vi "SUMMER SUNDAY BYTE[1].vi"() -> ()   [LabVIEW 2009]
uses:
  <vilib>/ULx/Create Channel.llb/ULx Create Channel (AI-Voltage-Basic).vi
  <vilib>/ULx/Read.llb/ULx Read (Analog DBL 1Chan 1Samp).vi
panel:
  out "POWER":bool
  out "data":dbl format="%_6g"
  out "xray":bool caption="BitValue"
  out "ENERGY LEVEL":dbl(knob) scale=0.0..15.0
  out "x*y":dbl
  out "Beam Pot":dbl format="%_6g"
  out "READY 2":bool
  out "DUMP":bool
  out "POWER":bool
  out "?":bool
  out "?":bool
  out "?":bool
  out "?":bool
  out "?":bool
  out "?":bool
  out "?":bool
  out "?":bool
  out "?":bool
  out "?":bool
  out "OPEN":bool
  out "CLOSED":bool
  out "READY":bool
  out "FAULT":bool
  out "MAGNET FORCE":dbl(slide) scale=0.0..10.0
  out "READY":bool
  out "TEMPERATURE":dbl(slide) scale=0.0..10.0
  in  "stop":bool
  out "?":bool
  out "?":bool
  out "?":bool
  out "?":bool
  in  "FAULT":bool
  out "POWER":bool
  out "FLOW IN GPM":dbl(knob) scale=0.0..15.0
  # "USERS LAB AREA"
  # "BEAM STATUS"
  # "ROOM"
  # "XRAY"
  # "PUMP STATION"
  # "MAGNET STATUS"
  # "ORBIT"
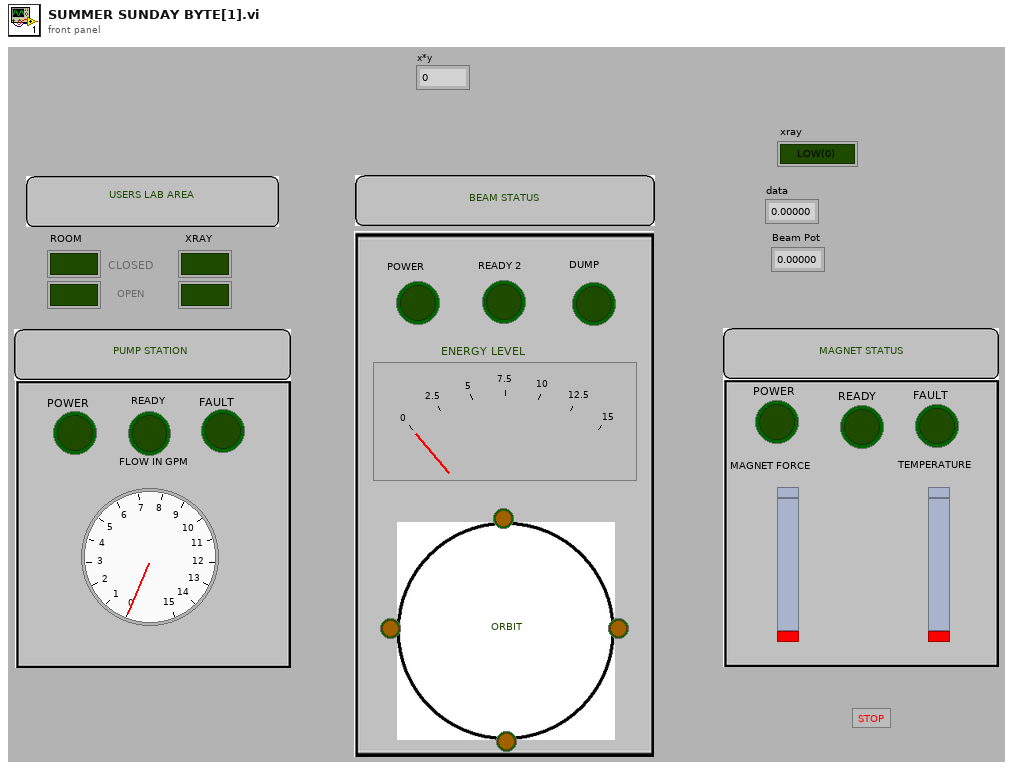
[diagram p1: front panel]
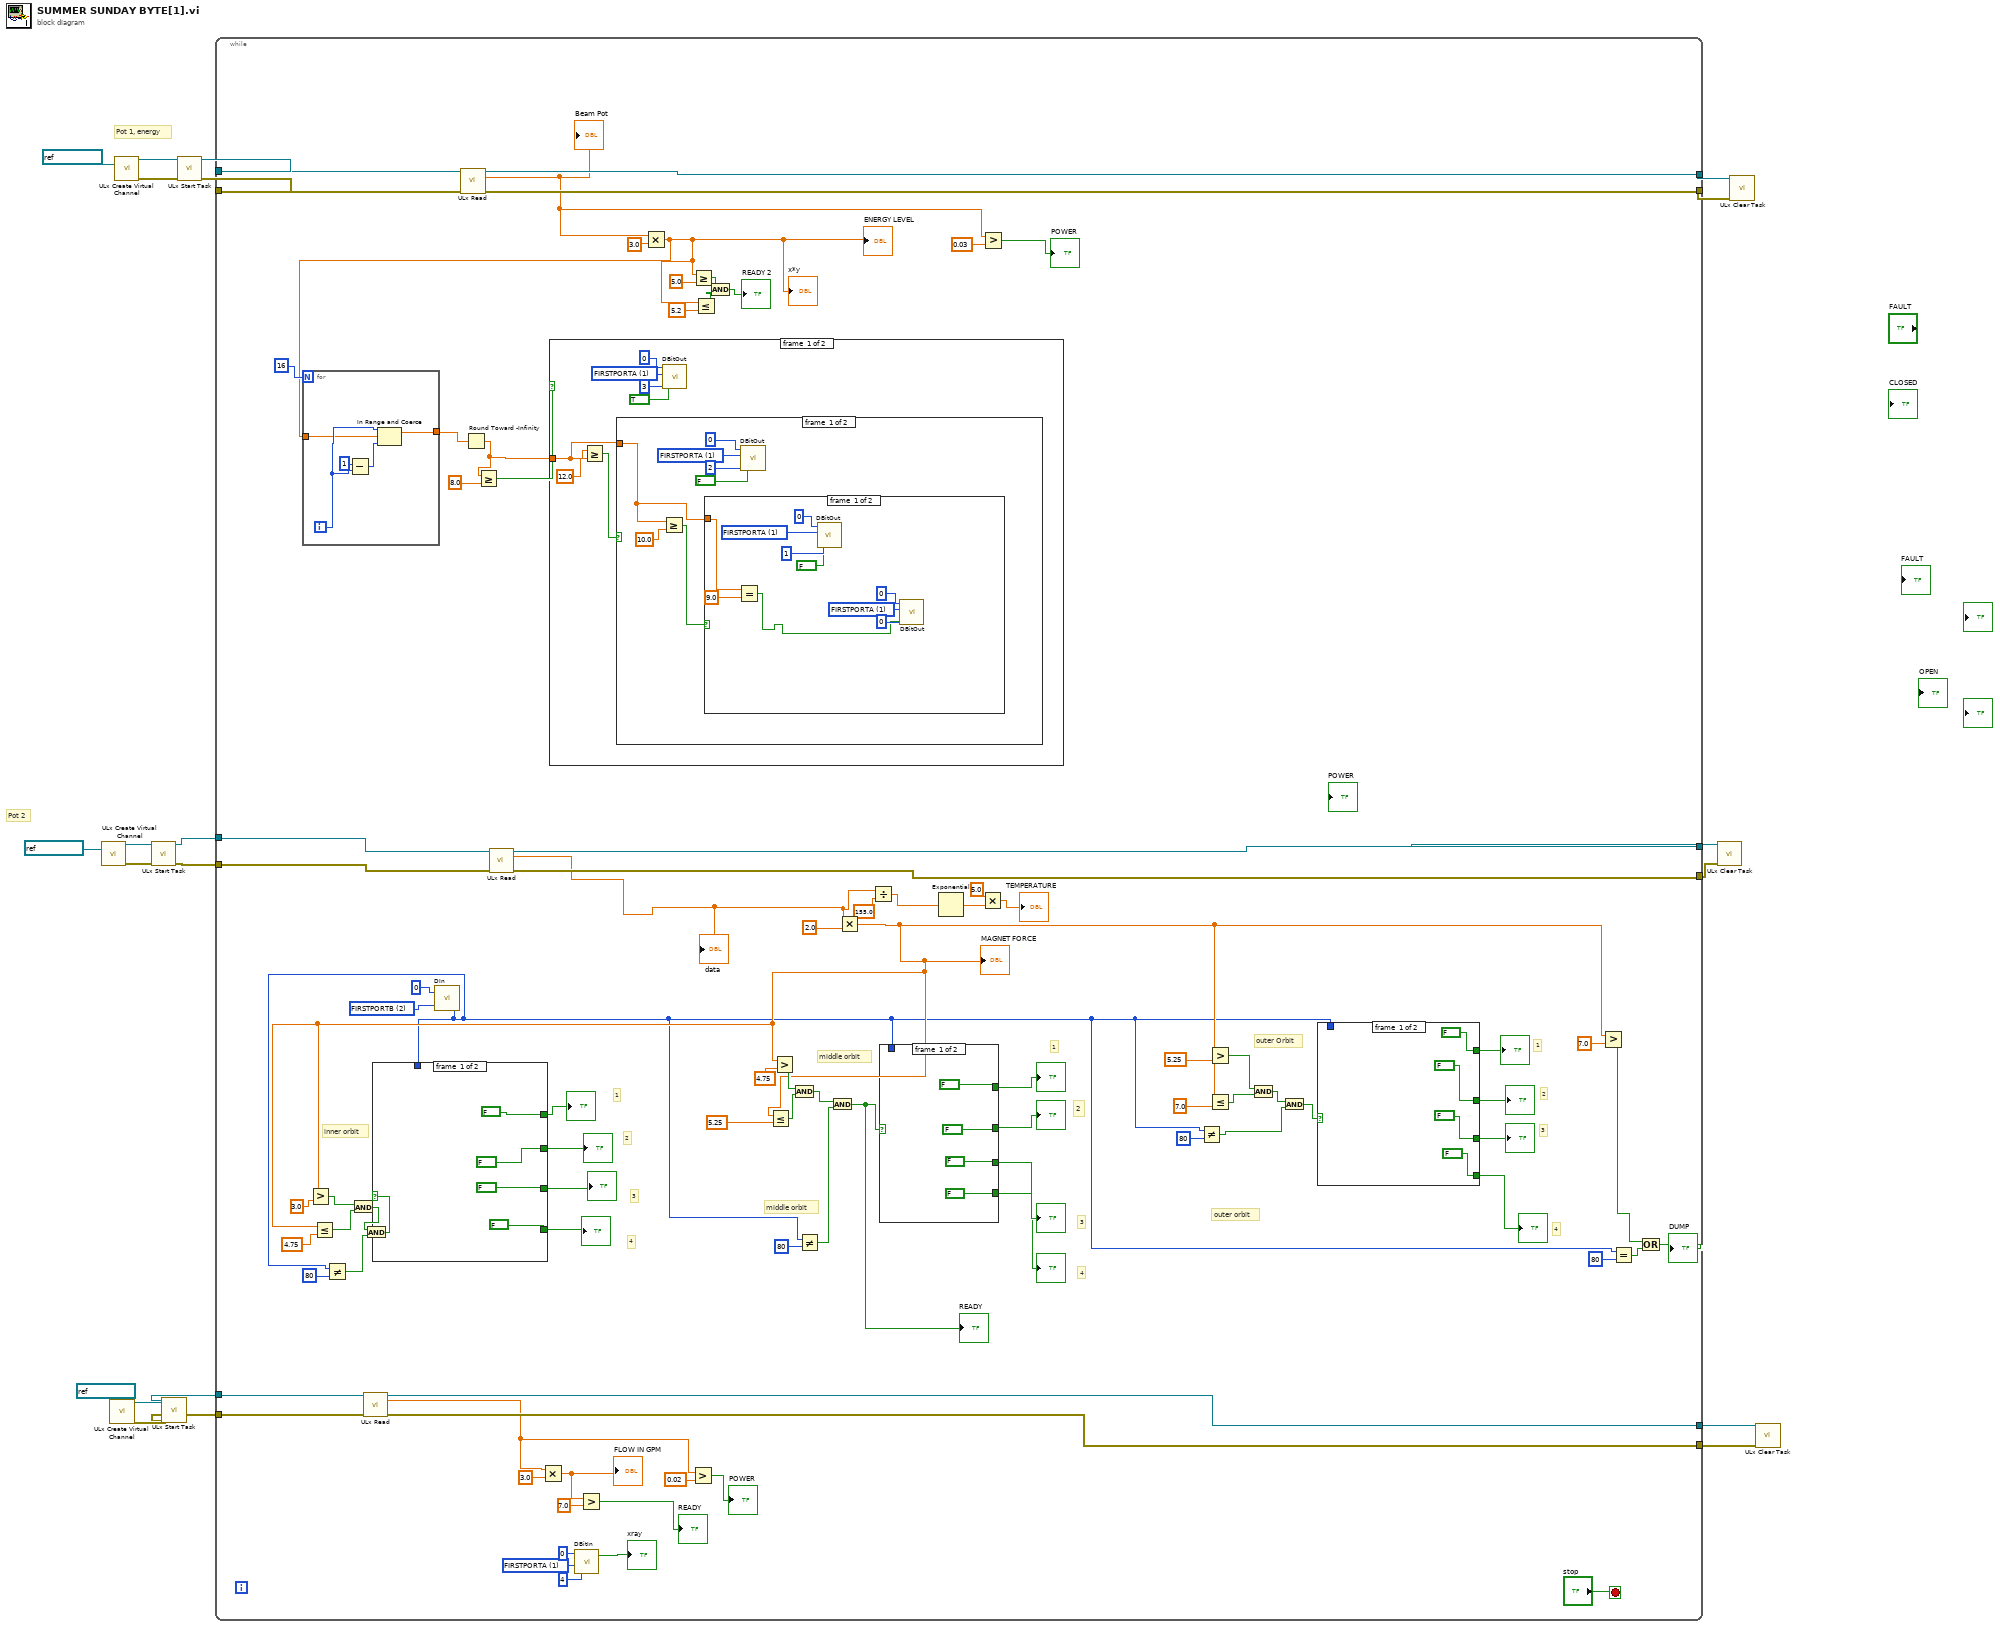
[diagram p0: block diagram]
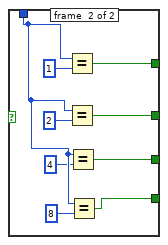
[diagram p2: hidden frame]
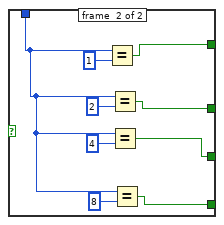
[diagram p3: hidden frame]
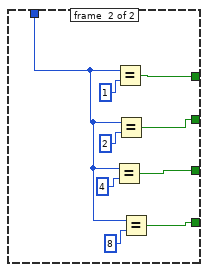
[diagram p4: hidden frame]
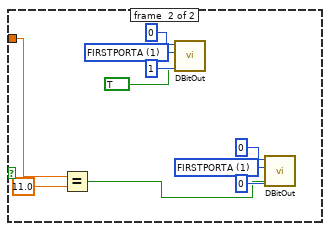
[diagram p5: hidden frame]
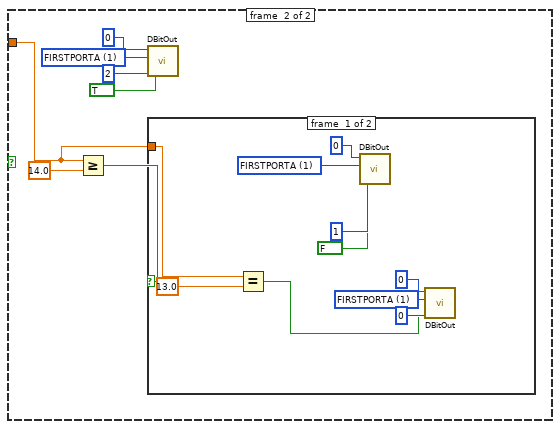
[diagram p6: hidden frame]
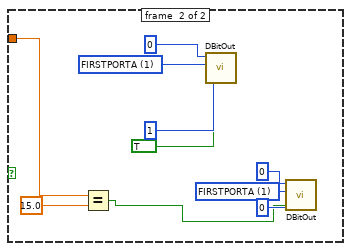
[diagram p7: hidden frame]
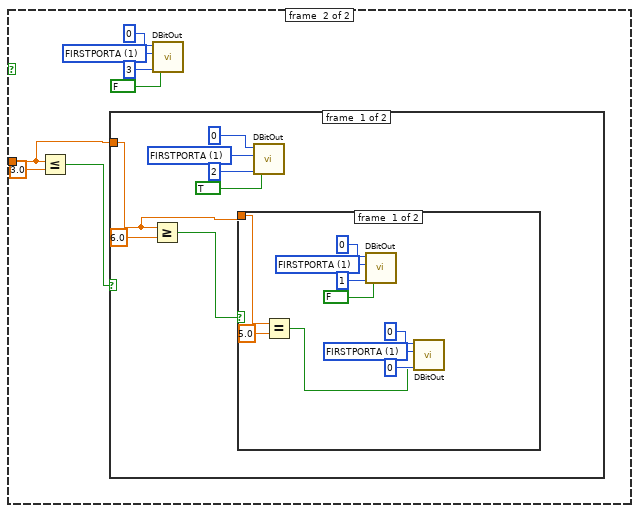
[diagram p8: hidden frame]
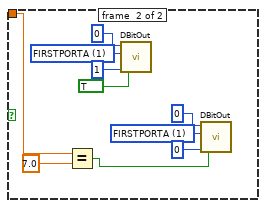
[diagram p9: hidden frame]
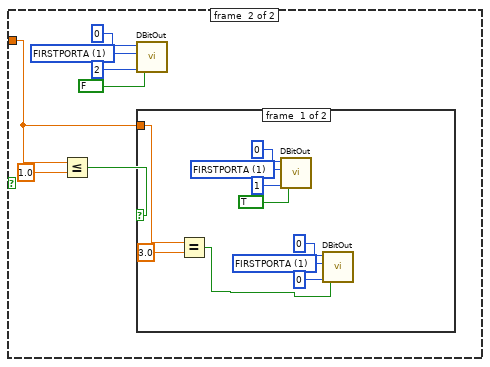
[diagram p10: hidden frame]
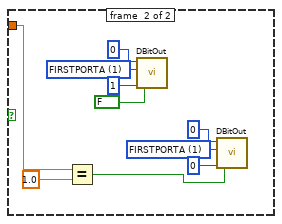
[diagram p11: hidden frame]
diagram:
  # "Pot 2"
  # "Pot 1, energy"
  n1 = call-poly <vilib>:"ULx Create Virtual Channel.vi"("physical channels"=refnum<k21> "Dev0/Ai1") -> ("task out"=w15:refnum<k24>, "error out"=w14:errorcluster)  [unwired: 13 in]
  n2 = call-poly <vilib>:"ULx Create Virtual Channel.vi"("physical channels"=refnum<k21> "Dev0/Ai2") -> ("task out"=w7:refnum<k24>, "error out"=w6:errorcluster)  [unwired: 13 in]
  n3 = call-poly <vilib>:"ULx Create Virtual Channel.vi"("physical channels"=refnum<k21> "Dev0/Ai0") -> ("task out"=w21:refnum<k24>, "error out"=w20:errorcluster)  [unwired: 13 in]
  n4 = call <vilib>:"ULx Start Task.vi"("task in"=w15, "error in"=w14) -> ("task out"=w13:refnum<k24>, "error out"=w12:errorcluster)  [unwired: 12 in]
  n5 = call <vilib>:"ULx Start Task.vi"("task in"=w7, "error in"=w6) -> ("task out"=w5:refnum<k24>, "error out"=w4:errorcluster)  [unwired: 12 in]
  n6 = call <vilib>:"ULx Start Task.vi"("task in"=w21, "error in"=w20) -> ("task out"=w19:refnum<k24>, "error out"=w18:errorcluster)  [unwired: 12 in]
  n7 = while {
    tunnel: w19 -> [w111]
    tunnel: w18 -> [w110]
    tunnel: [w109] -> w17
    tunnel: [w108] -> w16
    tunnel: w13 -> [w101]
    tunnel: w12 -> [w100]
    tunnel: [w99] -> w11
    tunnel: [w98] -> w10
    tunnel: w5 -> [w48]
    tunnel: w4 -> [w47]
    tunnel: [w46] -> w2
    tunnel: [w45] -> w1
    stop <- "stop" stop-if-true
    w43 = 1 items=["AUXPORT", "FIRSTPORTA"] ("PortType")
    w72 = 2 items=["AUXPORT", "FIRSTPORTA", "FIRSTPORTB", "FIRSTPORTCL", "FIRSTPORTCH", "SECONDPORTA", "SECONDPORTB", "SECONDPORTCL", "SECONDPORTCH", "THIRDPORTA", "THIRDPORTB", "THIRDPORTCL", "THIRDPORTCH", "FOURTHPORTA", "FOURTHPORTB", "FOURTHPORTCL", "FOURTHPORTCH", "FIFTHPORTA", "FIFTHPORTB", "FIFTHPORTCL", "FIFTHPORTCH", "SIXTHPORTA", "SIXTHPORTB", "SIXTHPORTCL", "SIXTHPORTCH", "SEVENTHPORTA", "SEVENTHPORTB", "SEVENTHPORTCL", "SEVENTHPORTCH", "EIGTHPORTA", "EIGHTHPORTB", "EIGHTHPORTCL", "EIGHTHPORTCH"] ("PortNum")
    # "outer Orbit"
    # "middle orbit"
    # "4"
    # "3"
    # "2"
    # "1"
    # "1"
    # "2"
    # "3"
    # "4"
    # "4"
    # "3"
    # "2"
    # "1"
    # "outer orbit"
    # "inner orbit"
    # "middle orbit"
    n8 = call-poly <vilib>:"ULx Read.vi"("task in"=w48, "error in"=w47) -> ("task out"=w46:refnum<k24>, "data"=w33:dbl, "error out"=w45:errorcluster)  [unwired: 11 in]
    n9 = call <menus>:"DIn.VI"("PortNum"=w72, "BoardNum"=u32 0) -> ("DataValue"=w60:i16)  [unwired: 1 out]
    n10 = Not Equal?(x=w60, y=i16 80) -> (x != y?=w84:bool)
    n11 = call-poly <vilib>:"ULx Read.vi"("task in"=w111, "error in"=w110) -> ("task out"=w109:refnum<k24>, "data"=w36:dbl, "error out"=w108:errorcluster)  [unwired: 11 in]
    "Beam Pot" <- w36
    n12 = call-poly <vilib>:"ULx Read.vi"("task in"=w101, "error in"=w100) -> ("task out"=w99:refnum<k24>, "data"=w34:dbl, "error out"=w98:errorcluster)  [unwired: 11 in]
    "data" <- w34
    n13 = Multiply(x=w33, y=3.0) -> (x*y=w32:dbl)
    "FLOW IN GPM" <- w32
    n14 = call <menus>:"DBitIn.VI"("BitNum"=4, "PortType"=w43, "BoardNum"=u32 0) -> ("BitValue"=→"xray":bool)  [unwired: 1 out]
    n15 = Greater?(x=w32, y=7.0) -> (0:→"READY":bool)
    n16 = Multiply(x=w36, y=3.0) -> (x*y=w26:dbl)
    "x*y" <- w26
    "ENERGY LEVEL" <- w26
    n17 = for {
      N: 16 -> [_]
      tunnel: w26 -> [w275]
      tunnel: [w274] -> w105
      i -> [w277]
      n18 = Subtract(x=1, y=w277) -> (x-y=w278:i32)
      n19 = In Range and Coerce(upper limit=w277, x=w275, lower limit=w278) -> (coerced(x)=w274:dbl)  [unwired: 1 out]
    }
    n20 = Round Toward -Infinity(1:w105) -> (0:w102:dbl)
    n21 = Greater Or Equal?(x=w102, y=8.0) -> (x >= y?=w103:bool)
    n22 = case shown="False" w103 {
      tunnel: w102 -> [w152 w213]
      frame #0 {
        w157 = u32 1 items=["AUXPORT", "FIRSTPORTA"] ("PortType")
        n23 = Greater Or Equal?(x=w152, y=12.0) -> (x >= y?=w153:bool)
        n24 = case shown="True" w153 {
          tunnel: w152 -> [w159 w186]
          frame #0 {
            w164 = u32 1 items=["AUXPORT", "FIRSTPORTA"] ("PortType")
            n25 = Greater Or Equal?(x=w159, y=10.0) -> (x >= y?=w160:bool)
            n26 = case shown="True" w160 {
              tunnel: w159 -> [w171 w182]
              frame #0 {
                w169 = u32 1 items=["AUXPORT", "FIRSTPORTA"] ("PortType")
                w174 = u32 1 items=["AUXPORT", "FIRSTPORTA"] ("PortType")
                n27 = Equal?(x=w171, y=9.0) -> (x = y?=w166:bool)
                n28 = call <menus>:"DBitOut.VI"("BitValue"=FALSE, "BitNum"=u32 1, "PortType"=w174, "BoardNum"=u32 0) -> ()  [unwired: 1 out]
                n29 = call <menus>:"DBitOut.VI"("BitValue"=w166, "BitNum"=u32 0, "PortType"=w169, "BoardNum"=u32 0) -> ()  [unwired: 1 out]
              }
              frame #1 {
                w179 = u32 1 items=["AUXPORT", "FIRSTPORTA"] ("PortType")
                w184 = u32 1 items=["AUXPORT", "FIRSTPORTA"] ("PortType")
                n30 = Equal?(x=w182, y=11.0) -> (x = y?=w176:bool)
                n31 = call <menus>:"DBitOut.VI"("BitValue"=TRUE, "BitNum"=u32 1, "PortType"=w184, "BoardNum"=u32 0) -> ()  [unwired: 1 out]
                n32 = call <menus>:"DBitOut.VI"("BitValue"=w176, "BitNum"=u32 0, "PortType"=w179, "BoardNum"=u32 0) -> ()  [unwired: 1 out]
              }
            }
            n33 = call <menus>:"DBitOut.VI"("BitValue"=FALSE, "BitNum"=u32 2, "PortType"=w164, "BoardNum"=u32 0) -> ()  [unwired: 1 out]
          }
          frame #1 {
            w191 = u32 1 items=["AUXPORT", "FIRSTPORTA"] ("PortType")
            n34 = Greater Or Equal?(x=w186, y=14.0) -> (x >= y?=w187:bool)
            n35 = call <menus>:"DBitOut.VI"("BitValue"=TRUE, "BitNum"=u32 2, "PortType"=w191, "BoardNum"=u32 0) -> ()  [unwired: 1 out]
            n36 = case shown="False" w187 {
              tunnel: w186 -> [w198 w208]
              frame #0 {
                w196 = u32 1 items=["AUXPORT", "FIRSTPORTA"] ("PortType")
                w201 = u32 1 items=["AUXPORT", "FIRSTPORTA"] ("PortType")
                n37 = Equal?(x=w198, y=13.0) -> (x = y?=w193:bool)
                n38 = call <menus>:"DBitOut.VI"("BitValue"=FALSE, "BitNum"=u32 1, "PortType"=w201, "BoardNum"=u32 0) -> ()  [unwired: 1 out]
                n39 = call <menus>:"DBitOut.VI"("BitValue"=w193, "BitNum"=u32 0, "PortType"=w196, "BoardNum"=u32 0) -> ()  [unwired: 1 out]
              }
              frame #1 {
                w206 = u32 1 items=["AUXPORT", "FIRSTPORTA"] ("PortType")
                w211 = u32 1 items=["AUXPORT", "FIRSTPORTA"] ("PortType")
                n40 = Equal?(x=w208, y=15.0) -> (x = y?=w203:bool)
                n41 = call <menus>:"DBitOut.VI"("BitValue"=TRUE, "BitNum"=u32 1, "PortType"=w211, "BoardNum"=u32 0) -> ()  [unwired: 1 out]
                n42 = call <menus>:"DBitOut.VI"("BitValue"=w203, "BitNum"=u32 0, "PortType"=w206, "BoardNum"=u32 0) -> ()  [unwired: 1 out]
              }
            }
          }
        }
        n43 = call <menus>:"DBitOut.VI"("BitValue"=TRUE, "BitNum"=u32 3, "PortType"=w157, "BoardNum"=u32 0) -> ()  [unwired: 1 out]
      }
      frame #1 {
        w218 = u32 1 items=["AUXPORT", "FIRSTPORTA"] ("PortType")
        n44 = Less Or Equal?(x=w213, y=3.0) -> (x <= y?=w214:bool)
        n45 = case shown="False" w214 {
          tunnel: w213 -> [w220 w247]
          frame #0 {
            w225 = u32 1 items=["AUXPORT", "FIRSTPORTA"] ("PortType")
            n46 = Greater Or Equal?(x=w220, y=6.0) -> (x >= y?=w221:bool)
            n47 = case shown="False" w221 {
              tunnel: w220 -> [w229 w242]
              frame #0 {
                w231 = u32 1 items=["AUXPORT", "FIRSTPORTA"] ("PortType")
                w235 = u32 1 items=["AUXPORT", "FIRSTPORTA"] ("PortType")
                n48 = Equal?(x=w229, y=5.0) -> (x = y?=w227:bool)
                n49 = call <menus>:"DBitOut.VI"("BitValue"=FALSE, "BitNum"=u32 1, "PortType"=w235, "BoardNum"=u32 0) -> ()  [unwired: 1 out]
                n50 = call <menus>:"DBitOut.VI"("BitValue"=w227, "BitNum"=u32 0, "PortType"=w231, "BoardNum"=u32 0) -> ()  [unwired: 1 out]
              }
              frame #1 {
                w239 = u32 1 items=["AUXPORT", "FIRSTPORTA"] ("PortType")
                w245 = u32 1 items=["AUXPORT", "FIRSTPORTA"] ("PortType")
                n51 = Equal?(x=w242, y=7.0) -> (x = y?=w237:bool)
                n52 = call <menus>:"DBitOut.VI"("BitValue"=TRUE, "BitNum"=u32 1, "PortType"=w245, "BoardNum"=u32 0) -> ()  [unwired: 1 out]
                n53 = call <menus>:"DBitOut.VI"("BitValue"=w237, "BitNum"=u32 0, "PortType"=w239, "BoardNum"=u32 0) -> ()  [unwired: 1 out]
              }
            }
            n54 = call <menus>:"DBitOut.VI"("BitValue"=TRUE, "BitNum"=u32 2, "PortType"=w225, "BoardNum"=u32 0) -> ()  [unwired: 1 out]
          }
          frame #1 {
            w252 = u32 1 items=["AUXPORT", "FIRSTPORTA"] ("PortType")
            n55 = Less Or Equal?(x=w247, y=1.0) -> (x <= y?=w248:bool)
            n56 = call <menus>:"DBitOut.VI"("BitValue"=FALSE, "BitNum"=u32 2, "PortType"=w252, "BoardNum"=u32 0) -> ()  [unwired: 1 out]
            n57 = case shown="True" w248 {
              tunnel: w247 -> [w259 w269]
              frame #0 {
                w256 = u32 1 items=["AUXPORT", "FIRSTPORTA"] ("PortType")
                w262 = u32 1 items=["AUXPORT", "FIRSTPORTA"] ("PortType")
                n58 = Equal?(x=w259, y=3.0) -> (x = y?=w254:bool)
                n59 = call <menus>:"DBitOut.VI"("BitValue"=TRUE, "BitNum"=u32 1, "PortType"=w262, "BoardNum"=u32 0) -> ()  [unwired: 1 out]
                n60 = call <menus>:"DBitOut.VI"("BitValue"=w254, "BitNum"=u32 0, "PortType"=w256, "BoardNum"=u32 0) -> ()  [unwired: 1 out]
              }
              frame #1 {
                w266 = u32 1 items=["AUXPORT", "FIRSTPORTA"] ("PortType")
                w272 = u32 1 items=["AUXPORT", "FIRSTPORTA"] ("PortType")
                n61 = Equal?(x=w269, y=1.0) -> (x = y?=w264:bool)
                n62 = call <menus>:"DBitOut.VI"("BitValue"=FALSE, "BitNum"=u32 1, "PortType"=w272, "BoardNum"=u32 0) -> ()  [unwired: 1 out]
                n63 = call <menus>:"DBitOut.VI"("BitValue"=w264, "BitNum"=u32 0, "PortType"=w266, "BoardNum"=u32 0) -> ()  [unwired: 1 out]
              }
            }
          }
        }
        n64 = call <menus>:"DBitOut.VI"("BitValue"=FALSE, "BitNum"=u32 3, "PortType"=w218, "BoardNum"=u32 0) -> ()  [unwired: 1 out]
      }
    }
    n65 = Greater?(x=w33, y=0.02) -> (0:→"POWER":bool)
    n66 = Greater Or Equal?(x=w26, y=5.0) -> (x >= y?=w23:bool)
    n67 = Less Or Equal?(x=w26, y=5.2) -> (x <= y?=w22:bool)
    n68 = And(x=w23, y=w22) -> (x .and. y?=→"READY 2":bool)
    n69 = Not Equal?(x=w60, y=i16 80) -> (x != y?=w68:bool)
    n70 = Multiply(x=w34, y=2.0) -> (x*y=w77:dbl)
    "MAGNET FORCE" <- w77
    n71 = Greater?(x=w77, y=3.0) -> (0:w94:bool)
    n72 = Less Or Equal?(x=w77, y=4.75) -> (x <= y?=w95:bool)
    n73 = And(x=w94, y=w95) -> (x .and. y?=w86:bool)
    n74 = And(x=w86, y=w84) -> (x .and. y?=w85:bool)
    n75 = case shown="True" w85 {
      tunnel: [FALSE w146] -> w56
      tunnel: [FALSE w145] -> w57
      tunnel: [FALSE w144] -> w54
      tunnel: [FALSE w143] -> w55
      tunnel: w60 -> [_ w151]
      frame #0 {
      }
      frame #1 {
        n76 = Equal?(x=w151, y=i16 4) -> (x = y?=w144:bool)
        n77 = Equal?(x=w151, y=i16 1) -> (x = y?=w146:bool)
        n78 = Equal?(x=w151, y=i16 2) -> (x = y?=w145:bool)
        n79 = Equal?(x=w151, y=i16 8) -> (x = y?=w143:bool)
      }
    }
    "?" <- w57
    "?" <- w54
    "?" <- w55
    "?" <- w56
    n80 = Less Or Equal?(x=w77, y=5.25) -> (x <= y?=w91:bool)
    n81 = Greater?(x=w77, y=4.75) -> (0:w92:bool)
    n82 = And(x=w92, y=w91) -> (x .and. y?=w83:bool)
    n83 = And(x=w83, y=w68) -> (x .and. y?=w29:bool)
    "READY" <- w29
    n84 = Divide(x=w34, y=155.0) -> (x/y=w52:dbl)
    n85 = case shown="True" w29 {
      tunnel: [FALSE w125] -> w67
      tunnel: [FALSE w124] -> w66
      tunnel: [FALSE w123] -> w65
      tunnel: [FALSE w122] -> w64
      tunnel: w60 -> [_ w121]
      frame #0 {
      }
      frame #1 {
        n86 = Equal?(x=w121, y=i16 1) -> (x = y?=w125:bool)
        n87 = Equal?(x=w121, y=i16 2) -> (x = y?=w124:bool)
        n88 = Equal?(x=w121, y=i16 4) -> (x = y?=w123:bool)
        n89 = Equal?(x=w121, y=i16 8) -> (x = y?=w122:bool)
      }
    }
    "?" <- w67
    "?" <- w66
    "?" <- w65
    "?" <- w64
    n90 = Exponential(1:w52) -> (0:w51:dbl)
    n91 = Multiply(x=5.0, y=w51) -> (x*y=→"TEMPERATURE":dbl)
    n92 = Greater?(x=w36, y=0.03) -> (0:→"POWER":bool)
    n93 = Not Equal?(x=w60, y=i16 80) -> (x != y?=w62:bool)
    n94 = Greater?(x=w77, y=5.25) -> (0:w89:bool)
    n95 = Less Or Equal?(x=w77, y=7.0) -> (x <= y?=w88:bool)
    n96 = And(x=w89, y=w88) -> (x .and. y?=w75:bool)
    n97 = And(x=w75, y=w62) -> (x .and. y?=w74:bool)
    n98 = case shown="True" w74 {
      tunnel: [FALSE w130] -> w81
      tunnel: [FALSE w131] -> w80
      tunnel: [FALSE w132] -> w79
      tunnel: [FALSE w133] -> w78
      tunnel: w60 -> [_ w138]
      frame #0 {
      }
      frame #1 {
        n99 = Equal?(x=w138, y=i16 1) -> (x = y?=w133:bool)
        n100 = Equal?(x=w138, y=i16 2) -> (x = y?=w132:bool)
        n101 = Equal?(x=w138, y=i16 4) -> (x = y?=w131:bool)
        n102 = Equal?(x=w138, y=i16 8) -> (x = y?=w130:bool)
      }
    }
    "?" <- w78
    "?" <- w79
    "?" <- w80
    "?" <- w81
    n103 = Greater?(x=w77, y=7.0) -> (0:w76:bool)
    n104 = Equal?(x=w60, y=i16 80) -> (x = y?=w58:bool)
    n105 = Or(x=w76, y=w58) -> (x .or. y?=→"DUMP":bool)
  }
  n106 = call <vilib>:"ULx Clear Task.vi"("task in"=w11, "error in"=w10) -> ()  [unwired: 13 in, 1 out]
  n107 = call <vilib>:"ULx Clear Task.vi"("task in"=w17, "error in"=w16) -> ()  [unwired: 13 in, 1 out]
  n108 = call <vilib>:"ULx Clear Task.vi"("task in"=w2, "error in"=w1) -> ()  [unwired: 13 in, 1 out]
